vi "ExSubInitNOpenCam.vi"(0 "error in (no error)":errorcluster) -> (1 "Camera Handle":u32, 2 "error out":errorcluster)   [LabVIEW 2014]
panel:
  # "ExSubInitNOpenCam:\nThis is a SubVI which initializes the SITK(tm) toolkit\nand opens a camera. If successful it returns a \ncamera handle."
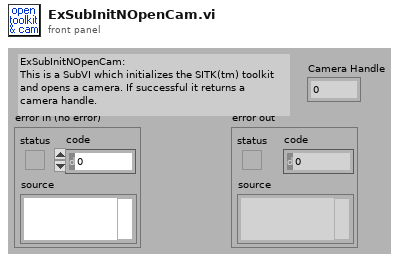
[diagram p1: front panel]
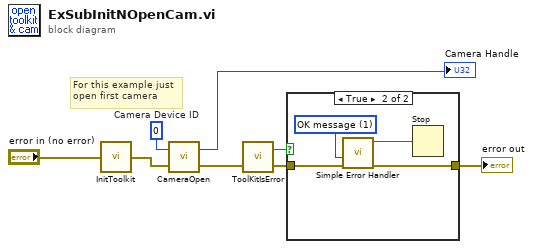
[diagram p0: block diagram]
diagram:
  w1 = u32 0  # Camera Device ID
  # "For this example just\nopen first camera"
  n1 = call <userlib>:"InitToolkit.vi"("error in"="error in (no error)") -> ("error out"=w7:errorcluster)
  n2 = call <userlib>:"CameraOpen.vi"("error in"=w7, "Camera Device ID"=w1) -> ("error out"=w5:errorcluster, "Camera Handle"=→"Camera Handle":u32)
  n3 = call <userlib>:"ToolKitIsError.vi"("error in"=w5) -> ("error out"=w3:errorcluster, "Error Flag"=w4:bool)  [unwired: 1 in]
  n4 = case shown="True" w4 {
    tunnel: w3 -> [w9 w13]
    tunnel: [w9 w11] -> w2
    frame False {
    }
    frame True {
      w10 = u16 1 items=["no dialog", "OK message", "continue or stop message"] ("type of dialog (OK msg:1)")
      n5 = call <vilib>:"Simple Error Handler.vi"("type of dialog (OK msg:1)"=w10, "error in (no error)"=w13) -> ("error?"=w12:bool, "error out"=w11:errorcluster)  [unwired: 3 in, 3 out]
      n6 = Stop(stop? (T)=w12) -> ()
    }
  }
  "error out" <- w2
